vi "Config Info Put.vi"(6 "PLC Comms":T2={"PLC boolean read Tags"={"AT glass position"={"Tag Name"="S060.PXI.Signals.PlltData.SN", "Network Path"="172.15.51.1,1,0", "use opc"=FALSE, "DataSocket Reference"={"CWDSLib._DCWDataSocket"=refnum, "CWDSLib._DCWData"=refnum, "OnDataUpdated"=0, "OnStatusUpdated"=0}}, "AT shade position"={"Tag Name"="S060.PXI.Signals.PlltData.SN", "Network Path"="172.15.51.1,1,0", "use opc"=FALSE, "DataSocket Reference"={"CWDSLib._DCWDataSocket"=refnum, "CWDSLib._DCWData"=refnum, "OnDataUpdated"=0, "OnStatusUpdated"=0}}, "AT in glass wand lower pos"={"Tag Name"="S060.PXI.Signals.PlltData.SN", "Network Path"="172.15.51.1,1,0", "use opc"=FALSE, "DataSocket Reference"={"CWDSLib._DCWDataSocket"=refnum, "CWDSLib._DCWData"=refnum, "OnDataUpdated"=0, "OnStatusUpdated"=0}}, "AT in glass wand up pos"={"Tag Name"="S060.PXI.Signals.PlltData.SN", "Network Path"="172.15.51.1,1,0", "use opc"=FALSE, "DataSocket Reference"={"CWDSLib._DCWDataSocket"=refnum, "CWDSLib._DCWData"=refnum, "OnDataUpdated"=0, "OnStatusUpdated"=0}}, "AT in sunshad wand lower pos"={"Tag Name"="S060.PXI.Signals.PlltData.SN", "Network Path"="172.15.51.1,1,0", "use opc"=FALSE, "DataSocket Reference"={"CWDSLib._DCWDataSocket"=refnum, "CWDSLib._DCWData"=refnum, "OnDataUpdated"=0, "OnStatusUpdated"=0}}, "AT in sunshad wand up pos"={"Tag Name"="S060.PXI.Signals.PlltData.SN", "Network Path"="172.15.51.1,1,0", "use opc"=FALSE, "DataSocket Reference"={"CWDSLib._DCWDataSocket"=refnum, "CWDSLib._DCWData"=refnum, "OnDataUpdated"=0, "OnStatusUpdated"=0}}, "AT in wand home pos"={"Tag Name"="S060.PXI.Signals.PlltData.SN", "Network Path"="172.15.51.1,1,0", "use opc"=FALSE, "DataSocket Reference"={"CWDSLib._DCWDataSocket"=refnum, "CWDSLib._DCWData"=refnum, "OnDataUpdated"=0, "OnStatusUpdated"=0}}, "LVDT's Extended"={"Tag Name"="S060.PXI.Signals.PlltData.SN", "Network Path"="172.15.51.1,1,0", "use opc"=FALSE, "DataSocket Reference"={"CWDSLib._DCWDataSocket"=refnum, "CWDSLib._DCWData"=refnum, "OnDataUpdated"=0, "OnStatusUpdated"=0}}, "bolt check 1"={"Tag Name"="S060.PXI.Signals.PlltData.SN", "Network Path"="172.15.51.1,1,0", "use opc"=FALSE, "DataSocket Reference"={"CWDSLib._DCWDataSocket"=refnum, "CWDSLib._DCWData"=refnum, "OnDataUpdated"=0, "OnStatusUpdated"=0}}, "bolt check 2"={"Tag Name"="S060.PXI.Signals.PlltData.SN", "Network Path"="172.15.51.1,1,0", "use opc"=FALSE, "DataSocket Reference"={"CWDSLib._DCWDataSocket"=refnum, "CWDSLib._DCWData"=refnum, "OnDataUpdated"=0, "OnStatusUpdated"=0}}, "bolt check 3"={"Tag Name"="S060.PXI.Signals.PlltData.SN", "Network Path"="172.15.51.1,1,0", "use opc"=FALSE, "DataSocket Reference"={"CWDSLib._DCWDataSocket"=refnum, "CWDSLib._DCWData"=refnum, "OnDataUpdated"=0, "OnStatusUpdated"=0}}, "bolt check 4"={"Tag Name"="S060.PXI.Signals.PlltData.SN", "Network Path"="172.15.51.1,1,0", "use opc"=FALSE, "DataSocket Reference"={"CWDSLib._DCWDataSocket"=refnum, "CWDSLib._DCWData"=refnum, "OnDataUpdated"=0, "OnStatusUpdated"=0}}, "bolt check 5"={"Tag Name"="S060.PXI.Signals.PlltData.SN", "Network Path"="172.15.51.1,1,0", "use opc"=FALSE, "DataSocket Reference"={"CWDSLib._DCWDataSocket"=refnum, "CWDSLib._DCWData"=refnum, "OnDataUpdated"=0, "OnStatusUpdated"=0}}, "bolt check 6"={"Tag Name"="S060.PXI.Signals.PlltData.SN", "Network Path"="172.15.51.1,1,0", "use opc"=FALSE, "DataSocket Reference"={"CWDSLib._DCWDataSocket"=refnum, "CWDSLib._DCWData"=refnum, "OnDataUpdated"=0, "OnStatusUpdated"=0}}, "bolt check 7"={"Tag Name"="S060.PXI.Signals.PlltData.SN", "Network Path"="172.15.51.1,1,0", "use opc"=FALSE, "DataSocket Reference"={"CWDSLib._DCWDataSocket"=refnum, "CWDSLib._DCWData"=refnum, "OnDataUpdated"=0, "OnStatusUpdated"=0}}, "bolt check 8"={"Tag Name"="S060.PXI.Signals.PlltData.SN", "Network Path"="172.15.51.1,1,0", "use opc"=FALSE, "DataSocket Reference"={"CWDSLib._DCWDataSocket"=refnum, "CWDSLib._DCWData"=refnum, "OnDataUpdated"=0, "OnStatusUpdated"=0}}, "start"={"Tag Name"="S060.PXI.Signals.PlltData.SN", "Network Path"="172.15.51.1,1,0", "use opc"=FALSE, "DataSocket Reference"={"CWDSLib._DCWDataSocket"=refnum, "CWDSLib._DCWData"=refnum, "OnDataUpdated"=0, "OnStatusUpdated"=0}}, "abort"={"Tag Name"="S060.PXI.Signals.PlltData.SN", "Network Path"="172.15.51.1,1,0", "use opc"=FALSE, "DataSocket Reference"={"CWDSLib._DCWDataSocket"=refnum, "CWDSLib._DCWData"=refnum, "OnDataUpdated"=0, "OnStatusUpdated"=0}}, "LVDT's Retracted"={"Tag Name"="S060.PXI.Signals.PlltData.SN", "Network Path"="172.15.51.1,1,0", "use opc"=FALSE, "DataSocket Reference"={"CWDSLib._DCWDataSocket"=refnum, "CWDSLib._DCWData"=refnum, "OnDataUpdated"=0, "OnStatusUpdated"=0}}, "manual barcode print"={"Tag Name"="S060.PXI.Signals.PlltData.SN", "Network Path"="172.15.51.1,1,0", "use opc"=FALSE, "DataSocket Reference"={"CWDSLib._DCWDataSocket"=refnum, "CWDSLib._DCWData"=refnum, "OnDataUpdated"=0, "OnStatusUpdated"=0}}, "ss servo at open"={"Tag Name"="S060.PXI.Signals.PlltData.SN", "Network Path"="172.15.51.1,1,0", "use opc"=FALSE, "DataSocket Reference"={"CWDSLib._DCWDataSocket"=refnum, "CWDSLib._DCWData"=refnum, "OnDataUpdated"=0, "OnStatusUpdated"=0}}, "ss servo at close"={"Tag Name"="S060.PXI.Signals.PlltData.SN", "Network Path"="172.15.51.1,1,0", "use opc"=FALSE, "DataSocket Reference"={"CWDSLib._DCWDataSocket"=refnum, "CWDSLib._DCWData"=refnum, "OnDataUpdated"=0, "OnStatusUpdated"=0}}, "ss servo opening"={"Tag Name"="S060.PXI.Signals.PlltData.SN", "Network Path"="172.15.51.1,1,0", "use opc"=FALSE, "DataSocket Reference"={"CWDSLib._DCWDataSocket"=refnum, "CWDSLib._DCWData"=refnum, "OnDataUpdated"=0, "OnStatusUpdated"=0}}, "ss servo closing"={"Tag Name"="S060.PXI.Signals.PlltData.SN", "Network Path"="172.15.51.1,1,0", "use opc"=FALSE, "DataSocket Reference"={"CWDSLib._DCWDataSocket"=refnum, "CWDSLib._DCWData"=refnum, "OnDataUpdated"=0, "OnStatusUpdated"=0}}, "control slide at home"={"Tag Name"="S060.PXI.Signals.PlltData.SN", "Network Path"="172.15.51.1,1,0", "use opc"=FALSE, "DataSocket Reference"={"CWDSLib._DCWDataSocket"=refnum, "CWDSLib._DCWData"=refnum, "OnDataUpdated"=0, "OnStatusUpdated"=0}}, "control slide left good"={"Tag Name"="S060.PXI.Signals.PlltData.SN", "Network Path"="172.15.51.1,1,0", "use opc"=FALSE, "DataSocket Reference"={"CWDSLib._DCWDataSocket"=refnum, "CWDSLib._DCWData"=refnum, "OnDataUpdated"=0, "OnStatusUpdated"=0}}, "control slide left over stroke"={"Tag Name"="S060.PXI.Signals.PlltData.SN", "Network Path"="172.15.51.1,1,0", "use opc"=FALSE, "DataSocket Reference"={"CWDSLib._DCWDataSocket"=refnum, "CWDSLib._DCWData"=refnum, "OnDataUpdated"=0, "OnStatusUpdated"=0}}, "control slide right good"={"Tag Name"="S060.PXI.Signals.PlltData.SN", "Network Path"="172.15.51.1,1,0", "use opc"=FALSE, "DataSocket Reference"={"CWDSLib._DCWDataSocket"=refnum, "CWDSLib._DCWData"=refnum, "OnDataUpdated"=0, "OnStatusUpdated"=0}}, "control slide right over stroke"={"Tag Name"="S060.PXI.Signals.PlltData.SN", "Network Path"="172.15.51.1,1,0", "use opc"=FALSE, "DataSocket Reference"={"CWDSLib._DCWDataSocket"=refnum, "CWDSLib._DCWData"=refnum, "OnDataUpdated"=0, "OnStatusUpdated"=0}}, "wind deflector high speed pos"={"Tag Name"="S060.PXI.Signals.PlltData.SN", "Network Path"="172.15.51.1,1,0", "use opc"=FALSE, "DataSocket Reference"={"CWDSLib._DCWDataSocket"=refnum, "CWDSLib._DCWData"=refnum, "OnDataUpdated"=0, "OnStatusUpdated"=0}}, "wind deflector low speed pos"={"Tag Name"="S060.PXI.Signals.PlltData.SN", "Network Path"="172.15.51.1,1,0", "use opc"=FALSE, "DataSocket Reference"={"CWDSLib._DCWDataSocket"=refnum, "CWDSLib._DCWData"=refnum, "OnDataUpdated"=0, "OnStatusUpdated"=0}}, "AT VentPMACatHome"={"Tag Name"="S060.PXI.Signals.PlltData.SN", "Network Path"="172.15.51.1,1,0", "use opc"=FALSE, "DataSocket Reference"={"CWDSLib._DCWDataSocket"=refnum, "CWDSLib._DCWData"=refnum, "OnDataUpdated"=0, "OnStatusUpdated"=0}}, "AT VentPMACisExtend"={"Tag Name"="S060.PXI.Signals.PlltData.SN", "Network Path"="172.15.51.1,1,0", "use opc"=FALSE, "DataSocket Reference"={"CWDSLib._DCWDataSocket"=refnum, "CWDSLib._DCWData"=refnum, "OnDataUpdated"=0, "OnStatusUpdated"=0}}, "SS Barcode Scanner Bypassed"={"Tag Name"="S060.PXI.Signals.PlltData.SN", "Network Path"="172.15.51.1,1,0", "use opc"=FALSE, "DataSocket Reference"={"CWDSLib._DCWDataSocket"=refnum, "CWDSLib._DCWData"=refnum, "OnDataUpdated"=0, "OnStatusUpdated"=0}}, "Check Frame Barcode"={"Tag Name"="S060.PXI.Signals.PlltData.SN", "Network Path"="172.15.51.1,1,0", "use opc"=FALSE, "DataSocket Reference"={"CWDSLib._DCWDataSocket"=refnum, "CWDSLib._DCWData"=refnum, "OnDataUpdated"=0, "OnStatusUpdated"=0}}, "Z LVDTs Extended"={"Tag Name"="S060.PXI.Signals.PlltData.SN", "Network Path"="172.15.51.1,1,0", "use opc"=FALSE, "DataSocket Reference"={"CWDSLib._DCWDataSocket"=refnum, "CWDSLib._DCWData"=refnum, "OnDataUpdated"=0, "OnStatusUpdated"=0}}, "NVH Operator Pass"={"Tag Name"="S060.PXI.Signals.PlltData.SN", "Network Path"="172.15.51.1,1,0", "use opc"=FALSE, "DataSocket Reference"={"CWDSLib._DCWDataSocket"=refnum, "CWDSLib._DCWData"=refnum, "OnDataUpdated"=0, "OnStatusUpdated"=0}}, "NVH Operator Fail"={"Tag Name"="S060.PXI.Signals.PlltData.SN", "Network Path"="172.15.51.1,1,0", "use opc"=FALSE, "DataSocket Reference"={"CWDSLib._DCWDataSocket"=refnum, "CWDSLib._DCWData"=refnum, "OnDataUpdated"=0, "OnStatusUpdated"=0}}, "NVH Operator Express Glass Open"={"Tag Name"="S060.PXI.Signals.PlltData.SN", "Network Path"="172.15.51.1,1,0", "use opc"=FALSE, "DataSocket Reference"={"CWDSLib._DCWDataSocket"=refnum, "CWDSLib._DCWData"=refnum, "OnDataUpdated"=0, "OnStatusUpdated"=0}}, "NVH Operator Express Glass Close"={"Tag Name"="S060.PXI.Signals.PlltData.SN", "Network Path"="172.15.51.1,1,0", "use opc"=FALSE, "DataSocket Reference"={"CWDSLib._DCWDataSocket"=refnum, "CWDSLib._DCWData"=refnum, "OnDataUpdated"=0, "OnStatusUpdated"=0}}, "NVH Operator Express Rollo Open01"={"Tag Name"="S060.PXI.Signals.PlltData.SN", "Network Path"="172.15.51.1,1,0", "use opc"=FALSE, "DataSocket Reference"={"CWDSLib._DCWDataSocket"=refnum, "CWDSLib._DCWData"=refnum, "OnDataUpdated"=0, "OnStatusUpdated"=0}}, "NVH Operator Express Rollo Close01"={"Tag Name"="S060.PXI.Signals.PlltData.SN", "Network Path"="172.15.51.1,1,0", "use opc"=FALSE, "DataSocket Reference"={"CWDSLib._DCWDataSocket"=refnum, "CWDSLib._DCWData"=refnum, "OnDataUpdated"=0, "OnStatusUpdated"=0}}, "NVH Operator Express Rollo Open02"={"Tag Name"="S060.PXI.Signals.PlltData.SN", "Network Path"="172.15.51.1,1,0", "use opc"=FALSE, "DataSocket Reference"={"CWDSLib._DCWDataSocket"=refnum, "CWDSLib._DCWData"=refnum, "OnDataUpdated"=0, "OnStatusUpdated"=0}}, "NVH Operator Express Rollo Close02"={"Tag Name"="S060.PXI.Signals.PlltData.SN", "Network Path"="172.15.51.1,1,0", "use opc"=FALSE, "DataSocket Reference"={"CWDSLib._DCWDataSocket"=refnum, "CWDSLib._DCWData"=refnum, "OnDataUpdated"=0, "OnStatusUpdated"=0}}, "NVH Operator Vent Open Noise"={"Tag Name"="S060.PXI.Signals.PlltData.SN", "Network Path"="172.15.51.1,1,0", "use opc"=FALSE, "DataSocket Reference"={"CWDSLib._DCWDataSocket"=refnum, "CWDSLib._DCWData"=refnum, "OnDataUpdated"=0, "OnStatusUpdated"=0}}, "NVH Operator Vent Close Noise"={"Tag Name"="S060.PXI.Signals.PlltData.SN", "Network Path"="172.15.51.1,1,0", "use opc"=FALSE, "DataSocket Reference"={"CWDSLib._DCWDataSocket"=refnum, "CWDSLib._DCWData"=refnum, "OnDataUpdated"=0, "OnStatusUpdated"=0}}, "NVH Operator Sunshade Open Noise"={"Tag Name"="S060.PXI.Signals.PlltData.SN", "Network Path"="172.15.51.1,1,0", "use opc"=FALSE, "DataSocket Reference"={"CWDSLib._DCWDataSocket"=refnum, "CWDSLib._DCWData"=refnum, "OnDataUpdated"=0, "OnStatusUpdated"=0}}, "NVH Operator Sunshade Close Noise"={"Tag Name"="S060.PXI.Signals.PlltData.SN", "Network Path"="172.15.51.1,1,0", "use opc"=FALSE, "DataSocket Reference"={"CWDSLib._DCWDataSocket"=refnum, "CWDSLib._DCWData"=refnum, "OnDataUpdated"=0, "OnStatusUpdated"=0}}, "NVH Operator Glass Open Noise"={"Tag Name"="S060.PXI.Signals.PlltData.SN", "Network Path"="172.15.51.1,1,0", "use opc"=FALSE, "DataSocket Reference"={"CWDSLib._DCWDataSocket"=refnum, "CWDSLib._DCWData"=refnum, "OnDataUpdated"=0, "OnStatusUpdated"=0}}, "NVH Operator Glass Close Noise"={"Tag Name"="S060.PXI.Signals.PlltData.SN", "Network Path"="172.15.51.1,1,0", "use opc"=FALSE, "DataSocket Reference"={"CWDSLib._DCWDataSocket"=refnum, "CWDSLib._DCWData"=refnum, "OnDataUpdated"=0, "OnStatusUpdated"=0}}, "NVH Operator Finish"={"Tag Name"="S060.PXI.Signals.PlltData.SN", "Network Path"="172.15.51.1,1,0", "use opc"=FALSE, "DataSocket Reference"={"CWDSLib._DCWDataSocket"=refnum, "CWDSLib._DCWData"=refnum, "OnDataUpdated"=0, "OnStatusUpdated"=0}}, "NVH Operator Check"={"Tag Name"="S060.PXI.Signals.PlltData.SN", "Network Path"="172.15.51.1,1,0", "use opc"=FALSE, "DataSocket Reference"={"CWDSLib._DCWDataSocket"=refnum, "CWDSLib._DCWData"=refnum, "OnDataUpdated"=0, "OnStatusUpdated"=0}}, "windproof position"={"Tag Name"="S060.PXI.Signals.PlltData.SN", "Network Path"="172.15.51.1,1,0", "use opc"=FALSE, "DataSocket Reference"={"CWDSLib._DCWDataSocket"=refnum, "CWDSLib._DCWData"=refnum, "OnDataUpdated"=0, "OnStatusUpdated"=0}}, "NVH Operator Express Glass vent Open"={"Tag Name"="S060.PXI.Signals.PlltData.SN", "Network Path"="172.15.51.1,1,0", "use opc"=FALSE, "DataSocket Reference"={"CWDSLib._DCWDataSocket"=refnum, "CWDSLib._DCWData"=refnum, "OnDataUpdated"=0, "OnStatusUpdated"=0}}, "NVH Operator Express Glass Vent Close"={"Tag Name"="S060.PXI.Signals.PlltData.SN", "Network Path"="172.15.51.1,1,0", "use opc"=FALSE, "DataSocket Reference"={"CWDSLib._DCWDataSocket"=refnum, "CWDSLib._DCWData"=refnum, "OnDataUpdated"=0, "OnStatusUpdated"=0}}, "NVH Operator Re-do"={"Tag Name"="S060.PXI.Signals.PlltData.SN", "Network Path"="172.15.51.1,1,0", "use opc"=FALSE, "DataSocket Reference"={"CWDSLib._DCWDataSocket"=refnum, "CWDSLib._DCWData"=refnum, "OnDataUpdated"=0, "OnStatusUpdated"=0}}, "AT at vent ATS test pos"={"Tag Name"="S060.PXI.Signals.PlltData.SN", "Network Path"="172.15.51.1,1,0", "use opc"=FALSE, "DataSocket Reference"={"CWDSLib._DCWDataSocket"=refnum, "CWDSLib._DCWData"=refnum, "OnDataUpdated"=0, "OnStatusUpdated"=0}}, "AT at vent ATS Home pos"={"Tag Name"="S060.PXI.Signals.PlltData.SN", "Network Path"="172.15.51.1,1,0", "use opc"=FALSE, "DataSocket Reference"={"CWDSLib._DCWDataSocket"=refnum, "CWDSLib._DCWData"=refnum, "OnDataUpdated"=0, "OnStatusUpdated"=0}}, "Start Adjust LVDT"={"Tag Name"="S060.PXI.Signals.PlltData.SN", "Network Path"="172.15.51.1,1,0", "use opc"=FALSE, "DataSocket Reference"={"CWDSLib._DCWDataSocket"=refnum, "CWDSLib._DCWData"=refnum, "OnDataUpdated"=0, "OnStatusUpdated"=0}}, "Finish Adjust LVDT"={"Tag Name"="S060.PXI.Signals.PlltData.SN", "Network Path"="172.15.51.1,1,0", "use opc"=FALSE, "DataSocket Reference"={"CWDSLib._DCWDataSocket"=refnum, "CWDSLib._DCWData"=refnum, "OnDataUpdated"=0, "OnStatusUpdated"=0}}}, "PLC bool write Tags"={"AT set glass wand lower"={"Tag Name"="S060.PXI.Signals.PlltData.SN", "Network Path"="172.15.51.1,1,0", "use opc"=FALSE, "DataSocket Reference"={"CWDSLib._DCWDataSocket"=refnum, "CWDSLib._DCWData"=refnum, "OnDataUpdated"=0, "OnStatusUpdated"=0}}, "AT set sunshade wand lower"={"Tag Name"="S060.PXI.Signals.PlltData.SN", "Network Path"="172.15.51.1,1,0", "use opc"=FALSE, "DataSocket Reference"={"CWDSLib._DCWDataSocket"=refnum, "CWDSLib._DCWData"=refnum, "OnDataUpdated"=0, "OnStatusUpdated"=0}}, "AT set sunshade wand up"={"Tag Name"="S060.PXI.Signals.PlltData.SN", "Network Path"="172.15.51.1,1,0", "use opc"=FALSE, "DataSocket Reference"={"CWDSLib._DCWDataSocket"=refnum, "CWDSLib._DCWData"=refnum, "OnDataUpdated"=0, "OnStatusUpdated"=0}}, "AT set glass wand up"={"Tag Name"="S060.PXI.Signals.PlltData.SN", "Network Path"="172.15.51.1,1,0", "use opc"=FALSE, "DataSocket Reference"={"CWDSLib._DCWDataSocket"=refnum, "CWDSLib._DCWData"=refnum, "OnDataUpdated"=0, "OnStatusUpdated"=0}}, "AT set wand home pos"={"Tag Name"="S060.PXI.Signals.PlltData.SN", "Network Path"="172.15.51.1,1,0", "use opc"=FALSE, "DataSocket Reference"={"CWDSLib._DCWDataSocket"=refnum, "CWDSLib._DCWData"=refnum, "OnDataUpdated"=0, "OnStatusUpdated"=0}}, "Test Complete Pass"={"Tag Name"="S060.PXI.Signals.PlltData.SN", "Network Path"="172.15.51.1,1,0", "use opc"=FALSE, "DataSocket Reference"={"CWDSLib._DCWDataSocket"=refnum, "CWDSLib._DCWData"=refnum, "OnDataUpdated"=0, "OnStatusUpdated"=0}}, "Test Complete Fail"={"Tag Name"="S060.PXI.Signals.PlltData.SN", "Network Path"="172.15.51.1,1,0", "use opc"=FALSE, "DataSocket Reference"={"CWDSLib._DCWDataSocket"=refnum, "CWDSLib._DCWData"=refnum, "OnDataUpdated"=0, "OnStatusUpdated"=0}}, "Test Started"={"Tag Name"="S060.PXI.Signals.PlltData.SN", "Network Path"="172.15.51.1,1,0", "use opc"=FALSE, "DataSocket Reference"={"CWDSLib._DCWDataSocket"=refnum, "CWDSLib._DCWData"=refnum, "OnDataUpdated"=0, "OnStatusUpdated"=0}}, "Retract LVDT's"={"Tag Name"="S060.PXI.Signals.PlltData.SN", "Network Path"="172.15.51.1,1,0", "use opc"=FALSE, "DataSocket Reference"={"CWDSLib._DCWDataSocket"=refnum, "CWDSLib._DCWData"=refnum, "OnDataUpdated"=0, "OnStatusUpdated"=0}}, "Extend LVDT's"={"Tag Name"="S060.PXI.Signals.PlltData.SN", "Network Path"="172.15.51.1,1,0", "use opc"=FALSE, "DataSocket Reference"={"CWDSLib._DCWDataSocket"=refnum, "CWDSLib._DCWData"=refnum, "OnDataUpdated"=0, "OnStatusUpdated"=0}}, "ss servo open"={"Tag Name"="S060.PXI.Signals.PlltData.SN", "Network Path"="172.15.51.1,1,0", "use opc"=FALSE, "DataSocket Reference"={"CWDSLib._DCWDataSocket"=refnum, "CWDSLib._DCWData"=refnum, "OnDataUpdated"=0, "OnStatusUpdated"=0}}, "ss servo close"={"Tag Name"="S060.PXI.Signals.PlltData.SN", "Network Path"="172.15.51.1,1,0", "use opc"=FALSE, "DataSocket Reference"={"CWDSLib._DCWDataSocket"=refnum, "CWDSLib._DCWData"=refnum, "OnDataUpdated"=0, "OnStatusUpdated"=0}}, "control slide start"={"Tag Name"="S060.PXI.Signals.PlltData.SN", "Network Path"="172.15.51.1,1,0", "use opc"=FALSE, "DataSocket Reference"={"CWDSLib._DCWDataSocket"=refnum, "CWDSLib._DCWData"=refnum, "OnDataUpdated"=0, "OnStatusUpdated"=0}}, "control slide stop"={"Tag Name"="S060.PXI.Signals.PlltData.SN", "Network Path"="172.15.51.1,1,0", "use opc"=FALSE, "DataSocket Reference"={"CWDSLib._DCWDataSocket"=refnum, "CWDSLib._DCWData"=refnum, "OnDataUpdated"=0, "OnStatusUpdated"=0}}, "AT VentPMACHome"={"Tag Name"="S060.PXI.Signals.PlltData.SN", "Network Path"="172.15.51.1,1,0", "use opc"=FALSE, "DataSocket Reference"={"CWDSLib._DCWDataSocket"=refnum, "CWDSLib._DCWData"=refnum, "OnDataUpdated"=0, "OnStatusUpdated"=0}}, "AT VentPMACExtended"={"Tag Name"="S060.PXI.Signals.PlltData.SN", "Network Path"="172.15.51.1,1,0", "use opc"=FALSE, "DataSocket Reference"={"CWDSLib._DCWDataSocket"=refnum, "CWDSLib._DCWData"=refnum, "OnDataUpdated"=0, "OnStatusUpdated"=0}}, "Good Frame Barcode"={"Tag Name"="S060.PXI.Signals.PlltData.SN", "Network Path"="172.15.51.1,1,0", "use opc"=FALSE, "DataSocket Reference"={"CWDSLib._DCWDataSocket"=refnum, "CWDSLib._DCWData"=refnum, "OnDataUpdated"=0, "OnStatusUpdated"=0}}, "Bad Frame Barcode"={"Tag Name"="S060.PXI.Signals.PlltData.SN", "Network Path"="172.15.51.1,1,0", "use opc"=FALSE, "DataSocket Reference"={"CWDSLib._DCWDataSocket"=refnum, "CWDSLib._DCWData"=refnum, "OnDataUpdated"=0, "OnStatusUpdated"=0}}, "Extend Z LVDTS"={"Tag Name"="S060.PXI.Signals.PlltData.SN", "Network Path"="172.15.51.1,1,0", "use opc"=FALSE, "DataSocket Reference"={"CWDSLib._DCWDataSocket"=refnum, "CWDSLib._DCWData"=refnum, "OnDataUpdated"=0, "OnStatusUpdated"=0}}, "NVH SunRoof Moving"={"Tag Name"="S060.PXI.Signals.PlltData.SN", "Network Path"="172.15.51.1,1,0", "use opc"=FALSE, "DataSocket Reference"={"CWDSLib._DCWDataSocket"=refnum, "CWDSLib._DCWData"=refnum, "OnDataUpdated"=0, "OnStatusUpdated"=0}}, "NVH SunRoof Stop"={"Tag Name"="S060.PXI.Signals.PlltData.SN", "Network Path"="172.15.51.1,1,0", "use opc"=FALSE, "DataSocket Reference"={"CWDSLib._DCWDataSocket"=refnum, "CWDSLib._DCWData"=refnum, "OnDataUpdated"=0, "OnStatusUpdated"=0}}, "NVH Pass"={"Tag Name"="S060.PXI.Signals.PlltData.SN", "Network Path"="172.15.51.1,1,0", "use opc"=FALSE, "DataSocket Reference"={"CWDSLib._DCWDataSocket"=refnum, "CWDSLib._DCWData"=refnum, "OnDataUpdated"=0, "OnStatusUpdated"=0}}, "NVH Fail"={"Tag Name"="S060.PXI.Signals.PlltData.SN", "Network Path"="172.15.51.1,1,0", "use opc"=FALSE, "DataSocket Reference"={"CWDSLib._DCWDataSocket"=refnum, "CWDSLib._DCWData"=refnum, "OnDataUpdated"=0, "OnStatusUpdated"=0}}, "NVH Operator Express Glass Opened"={"Tag Name"="S060.PXI.Signals.PlltData.SN", "Network Path"="172.15.51.1,1,0", "use opc"=FALSE, "DataSocket Reference"={"CWDSLib._DCWDataSocket"=refnum, "CWDSLib._DCWData"=refnum, "OnDataUpdated"=0, "OnStatusUpdated"=0}}, "NVH Operator Express Glass Closed"={"Tag Name"="S060.PXI.Signals.PlltData.SN", "Network Path"="172.15.51.1,1,0", "use opc"=FALSE, "DataSocket Reference"={"CWDSLib._DCWDataSocket"=refnum, "CWDSLib._DCWData"=refnum, "OnDataUpdated"=0, "OnStatusUpdated"=0}}, "NVH Operator Express Rollo Opened01"={"Tag Name"="S060.PXI.Signals.PlltData.SN", "Network Path"="172.15.51.1,1,0", "use opc"=FALSE, "DataSocket Reference"={"CWDSLib._DCWDataSocket"=refnum, "CWDSLib._DCWData"=refnum, "OnDataUpdated"=0, "OnStatusUpdated"=0}}, "NVH Operator Express Rollo Closed01"={"Tag Name"="S060.PXI.Signals.PlltData.SN", "Network Path"="172.15.51.1,1,0", "use opc"=FALSE, "DataSocket Reference"={"CWDSLib._DCWDataSocket"=refnum, "CWDSLib._DCWData"=refnum, "OnDataUpdated"=0, "OnStatusUpdated"=0}}, "NVH Operator Express Rollo Opened02"={"Tag Name"="S060.PXI.Signals.PlltData.SN", "Network Path"="172.15.51.1,1,0", "use opc"=FALSE, "DataSocket Reference"={"CWDSLib._DCWDataSocket"=refnum, "CWDSLib._DCWData"=refnum, "OnDataUpdated"=0, "OnStatusUpdated"=0}}, "NVH Operator Pass"={"Tag Name"="S060.PXI.Signals.PlltData.SN", "Network Path"="172.15.51.1,1,0", "use opc"=FALSE, "DataSocket Reference"={"CWDSLib._DCWDataSocket"=refnum, "CWDSLib._DCWData"=refnum, "OnDataUpdated"=0, "OnStatusUpdated"=0}}, "NVH Operator Fail"={"Tag Name"="S060.PXI.Signals.PlltData.SN", "Network Path"="172.15.51.1,1,0", "use opc"=FALSE, "DataSocket Reference"={"CWDSLib._DCWDataSocket"=refnum, "CWDSLib._DCWData"=refnum, "OnDataUpdated"=0, "OnStatusUpdated"=0}}, "NVH Operator Check"={"Tag Name"="S060.PXI.Signals.PlltData.SN", "Network Path"="172.15.51.1,1,0", "use opc"=FALSE, "DataSocket Reference"={"CWDSLib._DCWDataSocket"=refnum, "CWDSLib._DCWData"=refnum, "OnDataUpdated"=0, "OnStatusUpdated"=0}}, "NVH Operator Vent Open Noise"={"Tag Name"="S060.PXI.Signals.PlltData.SN", "Network Path"="172.15.51.1,1,0", "use opc"=FALSE, "DataSocket Reference"={"CWDSLib._DCWDataSocket"=refnum, "CWDSLib._DCWData"=refnum, "OnDataUpdated"=0, "OnStatusUpdated"=0}}, "NVH Operator Vent Close Noise"={"Tag Name"="S060.PXI.Signals.PlltData.SN", "Network Path"="172.15.51.1,1,0", "use opc"=FALSE, "DataSocket Reference"={"CWDSLib._DCWDataSocket"=refnum, "CWDSLib._DCWData"=refnum, "OnDataUpdated"=0, "OnStatusUpdated"=0}}, "NVH Operator Sunshade Open Noise"={"Tag Name"="S060.PXI.Signals.PlltData.SN", "Network Path"="172.15.51.1,1,0", "use opc"=FALSE, "DataSocket Reference"={"CWDSLib._DCWDataSocket"=refnum, "CWDSLib._DCWData"=refnum, "OnDataUpdated"=0, "OnStatusUpdated"=0}}, "NVH Operator Sunshade Close Noise"={"Tag Name"="S060.PXI.Signals.PlltData.SN", "Network Path"="172.15.51.1,1,0", "use opc"=FALSE, "DataSocket Reference"={"CWDSLib._DCWDataSocket"=refnum, "CWDSLib._DCWData"=refnum, "OnDataUpdated"=0, "OnStatusUpdated"=0}}, "NVH Operator Glass Open Noise"={"Tag Name"="S060.PXI.Signals.PlltData.SN", "Network Path"="172.15.51.1,1,0", "use opc"=FALSE, "DataSocket Reference"={"CWDSLib._DCWDataSocket"=refnum, "CWDSLib._DCWData"=refnum, "OnDataUpdated"=0, "OnStatusUpdated"=0}}, "NVH Operator Glass Close Noise"={"Tag Name"="S060.PXI.Signals.PlltData.SN", "Network Path"="172.15.51.1,1,0", "use opc"=FALSE, "DataSocket Reference"={"CWDSLib._DCWDataSocket"=refnum, "CWDSLib._DCWData"=refnum, "OnDataUpdated"=0, "OnStatusUpdated"=0}}, "NVH Operator Finish"={"Tag Name"="S060.PXI.Signals.PlltData.SN", "Network Path"="172.15.51.1,1,0", "use opc"=FALSE, "DataSocket Reference"={"CWDSLib._DCWDataSocket"=refnum, "CWDSLib._DCWData"=refnum, "OnDataUpdated"=0, "OnStatusUpdated"=0}}, "Barcode01 OK"={"Tag Name"="S060.PXI.Signals.PlltData.SN", "Network Path"="172.15.51.1,1,0", "use opc"=FALSE, "DataSocket Reference"={"CWDSLib._DCWDataSocket"=refnum, "CWDSLib._DCWData"=refnum, "OnDataUpdated"=0, "OnStatusUpdated"=0}}, "Barcode02 OK"={"Tag Name"="S060.PXI.Signals.PlltData.SN", "Network Path"="172.15.51.1,1,0", "use opc"=FALSE, "DataSocket Reference"={"CWDSLib._DCWDataSocket"=refnum, "CWDSLib._DCWData"=refnum, "OnDataUpdated"=0, "OnStatusUpdated"=0}}, "AT set to Vent ATS Test Pos"={"Tag Name"="S060.PXI.Signals.PlltData.SN", "Network Path"="172.15.51.1,1,0", "use opc"=FALSE, "DataSocket Reference"={"CWDSLib._DCWDataSocket"=refnum, "CWDSLib._DCWData"=refnum, "OnDataUpdated"=0, "OnStatusUpdated"=0}}, "AT set to Vent ATS Home Pos"={"Tag Name"="S060.PXI.Signals.PlltData.SN", "Network Path"="172.15.51.1,1,0", "use opc"=FALSE, "DataSocket Reference"={"CWDSLib._DCWDataSocket"=refnum, "CWDSLib._DCWData"=refnum, "OnDataUpdated"=0, "OnStatusUpdated"=0}}, "Move LVDT Adjust Station"={"Tag Name"="S060.PXI.Signals.PlltData.SN", "Network Path"="172.15.51.1,1,0", "use opc"=FALSE, "DataSocket Reference"={"CWDSLib._DCWDataSocket"=refnum, "CWDSLib._DCWData"=refnum, "OnDataUpdated"=0, "OnStatusUpdated"=0}}}, "PLC string read Tags"={"Serial Number"={"Tag Name"="S060.PXI.Signals.PlltData.SN", "Network Path"="172.15.51.1,1,0", "use opc"=FALSE, "DataSocket Reference"={"CWDSLib._DCWDataSocket"=refnum, "CWDSLib._DCWData"=refnum, "OnDataUpdated"=0, "OnStatusUpdated"=0}}, "Pallet Number"={"Tag Name"="S060.PXI.Signals.PlltData.SN", "Network Path"="172.15.51.1,1,0", "use opc"=FALSE, "DataSocket Reference"={"CWDSLib._DCWDataSocket"=refnum, "CWDSLib._DCWData"=refnum, "OnDataUpdated"=0, "OnStatusUpdated"=0}}, "Inalfa Part Number"={"Tag Name"="S060.PXI.Signals.PlltData.SN", "Network Path"="172.15.51.1,1,0", "use opc"=FALSE, "DataSocket Reference"={"CWDSLib._DCWDataSocket"=refnum, "CWDSLib._DCWData"=refnum, "OnDataUpdated"=0, "OnStatusUpdated"=0}}, "Shade Color"={"Tag Name"="S060.PXI.Signals.PlltData.SN", "Network Path"="172.15.51.1,1,0", "use opc"=FALSE, "DataSocket Reference"={"CWDSLib._DCWDataSocket"=refnum, "CWDSLib._DCWData"=refnum, "OnDataUpdated"=0, "OnStatusUpdated"=0}}, "Model Type"={"Tag Name"="S060.PXI.Signals.PlltData.SN", "Network Path"="172.15.51.1,1,0", "use opc"=FALSE, "DataSocket Reference"={"CWDSLib._DCWDataSocket"=refnum, "CWDSLib._DCWData"=refnum, "OnDataUpdated"=0, "OnStatusUpdated"=0}}, "Customer Number"={"Tag Name"="S060.PXI.Signals.PlltData.SN", "Network Path"="172.15.51.1,1,0", "use opc"=FALSE, "DataSocket Reference"={"CWDSLib._DCWDataSocket"=refnum, "CWDSLib._DCWData"=refnum, "OnDataUpdated"=0, "OnStatusUpdated"=0}}, "Part History Number"={"Tag Name"="S060.PXI.Signals.PlltData.SN", "Network Path"="172.15.51.1,1,0", "use opc"=FALSE, "DataSocket Reference"={"CWDSLib._DCWDataSocket"=refnum, "CWDSLib._DCWData"=refnum, "OnDataUpdated"=0, "OnStatusUpdated"=0}}, "Shade 1 Barcode"={"Tag Name"="S060.PXI.Signals.PlltData.SN", "Network Path"="172.15.51.1,1,0", "use opc"=FALSE, "DataSocket Reference"={"CWDSLib._DCWDataSocket"=refnum, "CWDSLib._DCWData"=refnum, "OnDataUpdated"=0, "OnStatusUpdated"=0}}, "Shade 2 Barcode"={"Tag Name"="S060.PXI.Signals.PlltData.SN", "Network Path"="172.15.51.1,1,0", "use opc"=FALSE, "DataSocket Reference"={"CWDSLib._DCWDataSocket"=refnum, "CWDSLib._DCWData"=refnum, "OnDataUpdated"=0, "OnStatusUpdated"=0}}, "Manual Serial Number"={"Tag Name"="S060.PXI.Signals.PlltData.SN", "Network Path"="172.15.51.1,1,0", "use opc"=FALSE, "DataSocket Reference"={"CWDSLib._DCWDataSocket"=refnum, "CWDSLib._DCWData"=refnum, "OnDataUpdated"=0, "OnStatusUpdated"=0}}, "Manual Inalfa Part Number"={"Tag Name"="S060.PXI.Signals.PlltData.SN", "Network Path"="172.15.51.1,1,0", "use opc"=FALSE, "DataSocket Reference"={"CWDSLib._DCWDataSocket"=refnum, "CWDSLib._DCWData"=refnum, "OnDataUpdated"=0, "OnStatusUpdated"=0}}, "Manual Shade Color"={"Tag Name"="S060.PXI.Signals.PlltData.SN", "Network Path"="172.15.51.1,1,0", "use opc"=FALSE, "DataSocket Reference"={"CWDSLib._DCWDataSocket"=refnum, "CWDSLib._DCWData"=refnum, "OnDataUpdated"=0, "OnStatusUpdated"=0}}, "Manual Model Type"={"Tag Name"="S060.PXI.Signals.PlltData.SN", "Network Path"="172.15.51.1,1,0", "use opc"=FALSE, "DataSocket Reference"={"CWDSLib._DCWDataSocket"=refnum, "CWDSLib._DCWData"=refnum, "OnDataUpdated"=0, "OnStatusUpdated"=0}}, "Manual Customer Number"={"Tag Name"="S060.PXI.Signals.PlltData.SN", "Network Path"="172.15.51.1,1,0", "use opc"=FALSE, "DataSocket Reference"={"CWDSLib._DCWDataSocket"=refnum, "CWDSLib._DCWData"=refnum, "OnDataUpdated"=0, "OnStatusUpdated"=0}}, "Manual Part History Number"={"Tag Name"="S060.PXI.Signals.PlltData.SN", "Network Path"="172.15.51.1,1,0", "use opc"=FALSE, "DataSocket Reference"={"CWDSLib._DCWDataSocket"=refnum, "CWDSLib._DCWData"=refnum, "OnDataUpdated"=0, "OnStatusUpdated"=0}}}, "PLC string write Tags"={"barcode station error"={"Tag Name"="S060.PXI.Signals.PlltData.SN", "Network Path"="172.15.51.1,1,0", "use opc"=FALSE, "DataSocket Reference"={"CWDSLib._DCWDataSocket"=refnum, "CWDSLib._DCWData"=refnum, "OnDataUpdated"=0, "OnStatusUpdated"=0}}, "error message 0"={"Tag Name"="S060.PXI.Signals.PlltData.SN", "Network Path"="172.15.51.1,1,0", "use opc"=FALSE, "DataSocket Reference"={"CWDSLib._DCWDataSocket"=refnum, "CWDSLib._DCWData"=refnum, "OnDataUpdated"=0, "OnStatusUpdated"=0}}, "error message 1"={"Tag Name"="S060.PXI.Signals.PlltData.SN", "Network Path"="172.15.51.1,1,0", "use opc"=FALSE, "DataSocket Reference"={"CWDSLib._DCWDataSocket"=refnum, "CWDSLib._DCWData"=refnum, "OnDataUpdated"=0, "OnStatusUpdated"=0}}, "error message 2"={"Tag Name"="S060.PXI.Signals.PlltData.SN", "Network Path"="172.15.51.1,1,0", "use opc"=FALSE, "DataSocket Reference"={"CWDSLib._DCWDataSocket"=refnum, "CWDSLib._DCWData"=refnum, "OnDataUpdated"=0, "OnStatusUpdated"=0}}, "error message 3"={"Tag Name"="S060.PXI.Signals.PlltData.SN", "Network Path"="172.15.51.1,1,0", "use opc"=FALSE, "DataSocket Reference"={"CWDSLib._DCWDataSocket"=refnum, "CWDSLib._DCWData"=refnum, "OnDataUpdated"=0, "OnStatusUpdated"=0}}}, "use opc"=FALSE, "PLC/OPC Path"=""} {"PLC string write Tags"."error message 3"."DataSocket Reference"."OnStatusUpdated" format="%.0x"; "PLC string write Tags"."error message 3"."DataSocket Reference"."OnDataUpdated" format="%.0x"; "PLC string write Tags"."error message 2"."DataSocket Reference"."OnStatusUpdated" format="%.0x"; "PLC string write Tags"."error message 2"."DataSocket Reference"."OnDataUpdated" format="%.0x"; "PLC string write Tags"."error message 1"."DataSocket Reference"."OnStatusUpdated" format="%.0x"; "PLC string write Tags"."error message 1"."DataSocket Reference"."OnDataUpdated" format="%.0x"; "PLC string write Tags"."error message 0"."DataSocket Reference"."OnStatusUpdated" format="%.0x"; "PLC string write Tags"."error message 0"."DataSocket Reference"."OnDataUpdated" format="%.0x"; "PLC string write Tags"."barcode station error"."DataSocket Reference"."OnStatusUpdated" format="%.0x"; "PLC string write Tags"."barcode station error"."DataSocket Reference"."OnDataUpdated" format="%.0x"; "PLC string read Tags"."Manual Part History Number"."DataSocket Reference"."OnStatusUpdated" format="%.0x"; "PLC string read Tags"."Manual Part History Number"."DataSocket Reference"."OnDataUpdated" format="%.0x"; "PLC string read Tags"."Manual Customer Number"."DataSocket Reference"."OnStatusUpdated" format="%.0x"; "PLC string read Tags"."Manual Customer Number"."DataSocket Reference"."OnDataUpdated" format="%.0x"; "PLC string read Tags"."Manual Model Type"."DataSocket Reference"."OnStatusUpdated" format="%.0x"; "PLC string read Tags"."Manual Model Type"."DataSocket Reference"."OnDataUpdated" format="%.0x"; "PLC string read Tags"."Manual Shade Color"."DataSocket Reference"."OnStatusUpdated" format="%.0x"; "PLC string read Tags"."Manual Shade Color"."DataSocket Reference"."OnDataUpdated" format="%.0x"; "PLC string read Tags"."Manual Inalfa Part Number"."DataSocket Reference"."OnStatusUpdated" format="%.0x"; "PLC string read Tags"."Manual Inalfa Part Number"."DataSocket Reference"."OnDataUpdated" format="%.0x"; "PLC string read Tags"."Manual Serial Number"."DataSocket Reference"."OnStatusUpdated" format="%.0x"; "PLC string read Tags"."Manual Serial Number"."DataSocket Reference"."OnDataUpdated" format="%.0x"; "PLC string read Tags"."Shade 2 Barcode"."DataSocket Reference"."OnStatusUpdated" format="%.0x"; "PLC string read Tags"."Shade 2 Barcode"."DataSocket Reference"."OnDataUpdated" format="%.0x"; "PLC string read Tags"."Shade 1 Barcode"."DataSocket Reference"."OnStatusUpdated" format="%.0x"; "PLC string read Tags"."Shade 1 Barcode"."DataSocket Reference"."OnDataUpdated" format="%.0x"; "PLC string read Tags"."Part History Number"."DataSocket Reference"."OnStatusUpdated" format="%.0x"; "PLC string read Tags"."Part History Number"."DataSocket Reference"."OnDataUpdated" format="%.0x"; "PLC string read Tags"."Customer Number"."DataSocket Reference"."OnStatusUpdated" format="%.0x"; "PLC string read Tags"."Customer Number"."DataSocket Reference"."OnDataUpdated" format="%.0x"; "PLC string read Tags"."Model Type"."DataSocket Reference"."OnStatusUpdated" format="%.0x"; "PLC string read Tags"."Model Type"."DataSocket Reference"."OnDataUpdated" format="%.0x"; "PLC string read Tags"."Shade Color"."DataSocket Reference"."OnStatusUpdated" format="%.0x"; "PLC string read Tags"."Shade Color"."DataSocket Reference"."OnDataUpdated" format="%.0x"; "PLC string read Tags"."Inalfa Part Number"."DataSocket Reference"."OnStatusUpdated" format="%.0x"; "PLC string read Tags"."Inalfa Part Number"."DataSocket Reference"."OnDataUpdated" format="%.0x"; "PLC string read Tags"."Pallet Number"."DataSocket Reference"."OnStatusUpdated" format="%.0x"; "PLC string read Tags"."Pallet Number"."DataSocket Reference"."OnDataUpdated" format="%.0x"; "PLC string read Tags"."Serial Number"."DataSocket Reference"."OnStatusUpdated" format="%.0x"; "PLC string read Tags"."Serial Number"."DataSocket Reference"."OnDataUpdated" format="%.0x"; "PLC bool write Tags"."Move LVDT Adjust Station"."DataSocket Reference"."OnStatusUpdated" format="%.0x"; "PLC bool write Tags"."Move LVDT Adjust Station"."DataSocket Reference"."OnDataUpdated" format="%.0x"; "PLC bool write Tags"."AT set to Vent ATS Home Pos"."DataSocket Reference"."OnStatusUpdated" format="%.0x"; "PLC bool write Tags"."AT set to Vent ATS Home Pos"."DataSocket Reference"."OnDataUpdated" format="%.0x"; "PLC bool write Tags"."AT set to Vent ATS Test Pos"."DataSocket Reference"."OnStatusUpdated" format="%.0x"; "PLC bool write Tags"."AT set to Vent ATS Test Pos"."DataSocket Reference"."OnDataUpdated" format="%.0x"; "PLC bool write Tags"."Barcode02 OK"."DataSocket Reference"."OnStatusUpdated" format="%.0x"; "PLC bool write Tags"."Barcode02 OK"."DataSocket Reference"."OnDataUpdated" format="%.0x"; "PLC bool write Tags"."Barcode01 OK"."DataSocket Reference"."OnStatusUpdated" format="%.0x"; "PLC bool write Tags"."Barcode01 OK"."DataSocket Reference"."OnDataUpdated" format="%.0x"; "PLC bool write Tags"."AT set glass wand up"."DataSocket Reference"."OnStatusUpdated" format="%.0x"; "PLC bool write Tags"."AT set glass wand up"."DataSocket Reference"."OnDataUpdated" format="%.0x"; "PLC bool write Tags"."AT set sunshade wand up"."DataSocket Reference"."OnStatusUpdated" format="%.0x"; "PLC bool write Tags"."AT set sunshade wand up"."DataSocket Reference"."OnDataUpdated" format="%.0x"; "PLC bool write Tags"."NVH Operator Finish"."DataSocket Reference"."OnStatusUpdated" format="%.0x"; "PLC bool write Tags"."NVH Operator Finish"."DataSocket Reference"."OnDataUpdated" format="%.0x"; "PLC bool write Tags"."NVH Operator Glass Close Noise"."DataSocket Reference"."OnStatusUpdated" format="%.0x"; "PLC bool write Tags"."NVH Operator Glass Close Noise"."DataSocket Reference"."OnDataUpdated" format="%.0x"; "PLC bool write Tags"."NVH Operator Glass Open Noise"."DataSocket Reference"."OnStatusUpdated" format="%.0x"; "PLC bool write Tags"."NVH Operator Glass Open Noise"."DataSocket Reference"."OnDataUpdated" format="%.0x"; "PLC bool write Tags"."NVH Operator Sunshade Close Noise"."DataSocket Reference"."OnStatusUpdated" format="%.0x"; "PLC bool write Tags"."NVH Operator Sunshade Close Noise"."DataSocket Reference"."OnDataUpdated" format="%.0x"; "PLC bool write Tags"."NVH Operator Sunshade Open Noise"."DataSocket Reference"."OnStatusUpdated" format="%.0x"; "PLC bool write Tags"."NVH Operator Sunshade Open Noise"."DataSocket Reference"."OnDataUpdated" format="%.0x"; "PLC bool write Tags"."NVH Operator Vent Close Noise"."DataSocket Reference"."OnStatusUpdated" format="%.0x"; "PLC bool write Tags"."NVH Operator Vent Close Noise"."DataSocket Reference"."OnDataUpdated" format="%.0x"; "PLC bool write Tags"."NVH Operator Vent Open Noise"."DataSocket Reference"."OnStatusUpdated" format="%.0x"; "PLC bool write Tags"."NVH Operator Vent Open Noise"."DataSocket Reference"."OnDataUpdated" format="%.0x"; "PLC bool write Tags"."NVH Operator Check"."DataSocket Reference"."OnStatusUpdated" format="%.0x"; "PLC bool write Tags"."NVH Operator Check"."DataSocket Reference"."OnDataUpdated" format="%.0x"; "PLC bool write Tags"."NVH Operator Fail"."DataSocket Reference"."OnStatusUpdated" format="%.0x"; "PLC bool write Tags"."NVH Operator Fail"."DataSocket Reference"."OnDataUpdated" format="%.0x"; "PLC bool write Tags"."NVH Operator Pass"."DataSocket Reference"."OnStatusUpdated" format="%.0x"; "PLC bool write Tags"."NVH Operator Pass"."DataSocket Reference"."OnDataUpdated" format="%.0x"; "PLC bool write Tags"."NVH Operator Express Rollo Opened02"."DataSocket Reference"."OnStatusUpdated" format="%.0x"; "PLC bool write Tags"."NVH Operator Express Rollo Opened02"."DataSocket Reference"."OnDataUpdated" format="%.0x"; "PLC bool write Tags"."NVH Operator Express Rollo Closed01"."DataSocket Reference"."OnStatusUpdated" format="%.0x"; "PLC bool write Tags"."NVH Operator Express Rollo Closed01"."DataSocket Reference"."OnDataUpdated" format="%.0x"; "PLC bool write Tags"."NVH Operator Express Rollo Opened01"."DataSocket Reference"."OnStatusUpdated" format="%.0x"; "PLC bool write Tags"."NVH Operator Express Rollo Opened01"."DataSocket Reference"."OnDataUpdated" format="%.0x"; "PLC bool write Tags"."NVH Operator Express Glass Closed"."DataSocket Reference"."OnStatusUpdated" format="%.0x"; "PLC bool write Tags"."NVH Operator Express Glass Closed"."DataSocket Reference"."OnDataUpdated" format="%.0x"; "PLC bool write Tags"."NVH Operator Express Glass Opened"."DataSocket Reference"."OnStatusUpdated" format="%.0x"; "PLC bool write Tags"."NVH Operator Express Glass Opened"."DataSocket Reference"."OnDataUpdated" format="%.0x"; "PLC bool write Tags"."NVH Fail"."DataSocket Reference"."OnStatusUpdated" format="%.0x"; "PLC bool write Tags"."NVH Fail"."DataSocket Reference"."OnDataUpdated" format="%.0x"; "PLC bool write Tags"."NVH Pass"."DataSocket Reference"."OnStatusUpdated" format="%.0x"; "PLC bool write Tags"."NVH Pass"."DataSocket Reference"."OnDataUpdated" format="%.0x"; "PLC bool write Tags"."NVH SunRoof Stop"."DataSocket Reference"."OnStatusUpdated" format="%.0x"; "PLC bool write Tags"."NVH SunRoof Stop"."DataSocket Reference"."OnDataUpdated" format="%.0x"; "PLC bool write Tags"."NVH SunRoof Moving"."DataSocket Reference"."OnStatusUpdated" format="%.0x"; "PLC bool write Tags"."NVH SunRoof Moving"."DataSocket Reference"."OnDataUpdated" format="%.0x"; "PLC bool write Tags"."Extend Z LVDTS"."DataSocket Reference"."OnStatusUpdated" format="%.0x"; "PLC bool write Tags"."Extend Z LVDTS"."DataSocket Reference"."OnDataUpdated" format="%.0x"; "PLC bool write Tags"."Bad Frame Barcode"."DataSocket Reference"."OnStatusUpdated" format="%.0x"; "PLC bool write Tags"."Bad Frame Barcode"."DataSocket Reference"."OnDataUpdated" format="%.0x"; "PLC bool write Tags"."Good Frame Barcode"."DataSocket Reference"."OnStatusUpdated" format="%.0x"; "PLC bool write Tags"."Good Frame Barcode"."DataSocket Reference"."OnDataUpdated" format="%.0x"; "PLC bool write Tags"."AT VentPMACExtended"."DataSocket Reference"."OnStatusUpdated" format="%.0x"; "PLC bool write Tags"."AT VentPMACExtended"."DataSocket Reference"."OnDataUpdated" format="%.0x"; "PLC bool write Tags"."AT VentPMACHome"."DataSocket Reference"."OnStatusUpdated" format="%.0x"; "PLC bool write Tags"."AT VentPMACHome"."DataSocket Reference"."OnDataUpdated" format="%.0x"; "PLC bool write Tags"."control slide stop"."DataSocket Reference"."OnStatusUpdated" format="%.0x"; "PLC bool write Tags"."control slide stop"."DataSocket Reference"."OnDataUpdated" format="%.0x"; "PLC bool write Tags"."control slide start"."DataSocket Reference"."OnStatusUpdated" format="%.0x"; "PLC bool write Tags"."control slide start"."DataSocket Reference"."OnDataUpdated" format="%.0x"; "PLC bool write Tags"."ss servo close"."DataSocket Reference"."OnStatusUpdated" format="%.0x"; "PLC bool write Tags"."ss servo close"."DataSocket Reference"."OnDataUpdated" format="%.0x"; "PLC bool write Tags"."ss servo open"."DataSocket Reference"."OnStatusUpdated" format="%.0x"; "PLC bool write Tags"."ss servo open"."DataSocket Reference"."OnDataUpdated" format="%.0x"; "PLC bool write Tags"."Extend LVDT's"."DataSocket Reference"."OnStatusUpdated" format="%.0x"; "PLC bool write Tags"."Extend LVDT's"."DataSocket Reference"."OnDataUpdated" format="%.0x"; "PLC bool write Tags"."Retract LVDT's"."DataSocket Reference"."OnStatusUpdated" format="%.0x"; "PLC bool write Tags"."Retract LVDT's"."DataSocket Reference"."OnDataUpdated" format="%.0x"; "PLC bool write Tags"."Test Started"."DataSocket Reference"."OnStatusUpdated" format="%.0x"; "PLC bool write Tags"."Test Started"."DataSocket Reference"."OnDataUpdated" format="%.0x"; "PLC bool write Tags"."Test Complete Fail"."DataSocket Reference"."OnStatusUpdated" format="%.0x"; "PLC bool write Tags"."Test Complete Fail"."DataSocket Reference"."OnDataUpdated" format="%.0x"; "PLC bool write Tags"."Test Complete Pass"."DataSocket Reference"."OnStatusUpdated" format="%.0x"; "PLC bool write Tags"."Test Complete Pass"."DataSocket Reference"."OnDataUpdated" format="%.0x"; "PLC bool write Tags"."AT set wand home pos"."DataSocket Reference"."OnStatusUpdated" format="%.0x"; "PLC bool write Tags"."AT set wand home pos"."DataSocket Reference"."OnDataUpdated" format="%.0x"; "PLC bool write Tags"."AT set sunshade wand lower"."DataSocket Reference"."OnStatusUpdated" format="%.0x"; "PLC bool write Tags"."AT set sunshade wand lower"."DataSocket Reference"."OnDataUpdated" format="%.0x"; "PLC bool write Tags"."AT set glass wand lower"."DataSocket Reference"."OnStatusUpdated" format="%.0x"; "PLC bool write Tags"."AT set glass wand lower"."DataSocket Reference"."OnDataUpdated" format="%.0x"; "PLC boolean read Tags"."AT in sunshad wand up pos"."DataSocket Reference"."OnStatusUpdated" format="%.0x"; "PLC boolean read Tags"."AT in sunshad wand up pos"."DataSocket Reference"."OnDataUpdated" format="%.0x"; "PLC boolean read Tags"."AT in glass wand up pos"."DataSocket Reference"."OnStatusUpdated" format="%.0x"; "PLC boolean read Tags"."AT in glass wand up pos"."DataSocket Reference"."OnDataUpdated" format="%.0x"; "PLC boolean read Tags"."Finish Adjust LVDT"."DataSocket Reference"."OnStatusUpdated" format="%.0x"; "PLC boolean read Tags"."Finish Adjust LVDT"."DataSocket Reference"."OnDataUpdated" format="%.0x"; "PLC boolean read Tags"."Start Adjust LVDT"."DataSocket Reference"."OnStatusUpdated" format="%.0x"; "PLC boolean read Tags"."Start Adjust LVDT"."DataSocket Reference"."OnDataUpdated" format="%.0x"; "PLC boolean read Tags"."AT at vent ATS Home pos"."DataSocket Reference"."OnStatusUpdated" format="%.0x"; "PLC boolean read Tags"."AT at vent ATS Home pos"."DataSocket Reference"."OnDataUpdated" format="%.0x"; "PLC boolean read Tags"."AT at vent ATS test pos"."DataSocket Reference"."OnStatusUpdated" format="%.0x"; "PLC boolean read Tags"."AT at vent ATS test pos"."DataSocket Reference"."OnDataUpdated" format="%.0x"; "PLC boolean read Tags"."NVH Operator Re-do"."DataSocket Reference"."OnStatusUpdated" format="%.0x"; "PLC boolean read Tags"."NVH Operator Re-do"."DataSocket Reference"."OnDataUpdated" format="%.0x"; "PLC boolean read Tags"."NVH Operator Express Glass Vent Close"."DataSocket Reference"."OnStatusUpdated" format="%.0x"; "PLC boolean read Tags"."NVH Operator Express Glass Vent Close"."DataSocket Reference"."OnDataUpdated" format="%.0x"; "PLC boolean read Tags"."NVH Operator Express Glass vent Open"."DataSocket Reference"."OnStatusUpdated" format="%.0x"; "PLC boolean read Tags"."NVH Operator Express Glass vent Open"."DataSocket Reference"."OnDataUpdated" format="%.0x"; "PLC boolean read Tags"."windproof position"."DataSocket Reference"."OnStatusUpdated" format="%.0x"; "PLC boolean read Tags"."windproof position"."DataSocket Reference"."OnDataUpdated" format="%.0x"; "PLC boolean read Tags"."NVH Operator Check"."DataSocket Reference"."OnStatusUpdated" format="%.0x"; "PLC boolean read Tags"."NVH Operator Check"."DataSocket Reference"."OnDataUpdated" format="%.0x"; "PLC boolean read Tags"."NVH Operator Finish"."DataSocket Reference"."OnStatusUpdated" format="%.0x"; "PLC boolean read Tags"."NVH Operator Finish"."DataSocket Reference"."OnDataUpdated" format="%.0x"; "PLC boolean read Tags"."NVH Operator Glass Close Noise"."DataSocket Reference"."OnStatusUpdated" format="%.0x"; "PLC boolean read Tags"."NVH Operator Glass Close Noise"."DataSocket Reference"."OnDataUpdated" format="%.0x"; "PLC boolean read Tags"."NVH Operator Glass Open Noise"."DataSocket Reference"."OnStatusUpdated" format="%.0x"; "PLC boolean read Tags"."NVH Operator Glass Open Noise"."DataSocket Reference"."OnDataUpdated" format="%.0x"; "PLC boolean read Tags"."NVH Operator Sunshade Close Noise"."DataSocket Reference"."OnStatusUpdated" format="%.0x"; "PLC boolean read Tags"."NVH Operator Sunshade Close Noise"."DataSocket Reference"."OnDataUpdated" format="%.0x"; "PLC boolean read Tags"."NVH Operator Sunshade Open Noise"."DataSocket Reference"."OnStatusUpdated" format="%.0x"; "PLC boolean read Tags"."NVH Operator Sunshade Open Noise"."DataSocket Reference"."OnDataUpdated" format="%.0x"; "PLC boolean read Tags"."NVH Operator Vent Close Noise"."DataSocket Reference"."OnStatusUpdated" format="%.0x"; "PLC boolean read Tags"."NVH Operator Vent Close Noise"."DataSocket Reference"."OnDataUpdated" format="%.0x"; "PLC boolean read Tags"."NVH Operator Vent Open Noise"."DataSocket Reference"."OnStatusUpdated" format="%.0x"; "PLC boolean read Tags"."NVH Operator Vent Open Noise"."DataSocket Reference"."OnDataUpdated" format="%.0x"; "PLC boolean read Tags"."NVH Operator Express Rollo Close02"."DataSocket Reference"."OnStatusUpdated" format="%.0x"; "PLC boolean read Tags"."NVH Operator Express Rollo Close02"."DataSocket Reference"."OnDataUpdated" format="%.0x"; "PLC boolean read Tags"."NVH Operator Express Rollo Open02"."DataSocket Reference"."OnStatusUpdated" format="%.0x"; "PLC boolean read Tags"."NVH Operator Express Rollo Open02"."DataSocket Reference"."OnDataUpdated" format="%.0x"; "PLC boolean read Tags"."NVH Operator Express Rollo Close01"."DataSocket Reference"."OnStatusUpdated" format="%.0x"; "PLC boolean read Tags"."NVH Operator Express Rollo Close01"."DataSocket Reference"."OnDataUpdated" format="%.0x"; "PLC boolean read Tags"."NVH Operator Express Rollo Open01"."DataSocket Reference"."OnStatusUpdated" format="%.0x"; "PLC boolean read Tags"."NVH Operator Express Rollo Open01"."DataSocket Reference"."OnDataUpdated" format="%.0x"; "PLC boolean read Tags"."NVH Operator Express Glass Close"."DataSocket Reference"."OnStatusUpdated" format="%.0x"; "PLC boolean read Tags"."NVH Operator Express Glass Close"."DataSocket Reference"."OnDataUpdated" format="%.0x"; "PLC boolean read Tags"."NVH Operator Express Glass Open"."DataSocket Reference"."OnStatusUpdated" format="%.0x"; "PLC boolean read Tags"."NVH Operator Express Glass Open"."DataSocket Reference"."OnDataUpdated" format="%.0x"; "PLC boolean read Tags"."NVH Operator Fail"."DataSocket Reference"."OnStatusUpdated" format="%.0x"; "PLC boolean read Tags"."NVH Operator Fail"."DataSocket Reference"."OnDataUpdated" format="%.0x"; "PLC boolean read Tags"."NVH Operator Pass"."DataSocket Reference"."OnStatusUpdated" format="%.0x"; "PLC boolean read Tags"."NVH Operator Pass"."DataSocket Reference"."OnDataUpdated" format="%.0x"; "PLC boolean read Tags"."Z LVDTs Extended"."DataSocket Reference"."OnStatusUpdated" format="%.0x"; "PLC boolean read Tags"."Z LVDTs Extended"."DataSocket Reference"."OnDataUpdated" format="%.0x"; "PLC boolean read Tags"."Check Frame Barcode"."DataSocket Reference"."OnStatusUpdated" format="%.0x"; "PLC boolean read Tags"."Check Frame Barcode"."DataSocket Reference"."OnDataUpdated" format="%.0x"; "PLC boolean read Tags"."SS Barcode Scanner Bypassed"."DataSocket Reference"."OnStatusUpdated" format="%.0x"; "PLC boolean read Tags"."SS Barcode Scanner Bypassed"."DataSocket Reference"."OnDataUpdated" format="%.0x"; "PLC boolean read Tags"."AT VentPMACisExtend"."DataSocket Reference"."OnStatusUpdated" format="%.0x"; "PLC boolean read Tags"."AT VentPMACisExtend"."DataSocket Reference"."OnDataUpdated" format="%.0x"; "PLC boolean read Tags"."AT VentPMACatHome"."DataSocket Reference"."OnStatusUpdated" format="%.0x"; "PLC boolean read Tags"."AT VentPMACatHome"."DataSocket Reference"."OnDataUpdated" format="%.0x"; "PLC boolean read Tags"."wind deflector low speed pos"."DataSocket Reference"."OnStatusUpdated" format="%.0x"; "PLC boolean read Tags"."wind deflector low speed pos"."DataSocket Reference"."OnDataUpdated" format="%.0x"; "PLC boolean read Tags"."wind deflector high speed pos"."DataSocket Reference"."OnStatusUpdated" format="%.0x"; "PLC boolean read Tags"."wind deflector high speed pos"."DataSocket Reference"."OnDataUpdated" format="%.0x"; "PLC boolean read Tags"."control slide right over stroke"."DataSocket Reference"."OnStatusUpdated" format="%.0x"; "PLC boolean read Tags"."control slide right over stroke"."DataSocket Reference"."OnDataUpdated" format="%.0x"; "PLC boolean read Tags"."control slide right good"."DataSocket Reference"."OnStatusUpdated" format="%.0x"; "PLC boolean read Tags"."control slide right good"."DataSocket Reference"."OnDataUpdated" format="%.0x"; "PLC boolean read Tags"."control slide left over stroke"."DataSocket Reference"."OnStatusUpdated" format="%.0x"; "PLC boolean read Tags"."control slide left over stroke"."DataSocket Reference"."OnDataUpdated" format="%.0x"; "PLC boolean read Tags"."control slide left good"."DataSocket Reference"."OnStatusUpdated" format="%.0x"; "PLC boolean read Tags"."control slide left good"."DataSocket Reference"."OnDataUpdated" format="%.0x"; "PLC boolean read Tags"."control slide at home"."DataSocket Reference"."OnStatusUpdated" format="%.0x"; "PLC boolean read Tags"."control slide at home"."DataSocket Reference"."OnDataUpdated" format="%.0x"; "PLC boolean read Tags"."ss servo closing"."DataSocket Reference"."OnStatusUpdated" format="%.0x"; "PLC boolean read Tags"."ss servo closing"."DataSocket Reference"."OnDataUpdated" format="%.0x"; "PLC boolean read Tags"."ss servo opening"."DataSocket Reference"."OnStatusUpdated" format="%.0x"; "PLC boolean read Tags"."ss servo opening"."DataSocket Reference"."OnDataUpdated" format="%.0x"; "PLC boolean read Tags"."ss servo at close"."DataSocket Reference"."OnStatusUpdated" format="%.0x"; "PLC boolean read Tags"."ss servo at close"."DataSocket Reference"."OnDataUpdated" format="%.0x"; "PLC boolean read Tags"."ss servo at open"."DataSocket Reference"."OnStatusUpdated" format="%.0x"; "PLC boolean read Tags"."ss servo at open"."DataSocket Reference"."OnDataUpdated" format="%.0x"; "PLC boolean read Tags"."manual barcode print"."DataSocket Reference"."OnStatusUpdated" format="%.0x"; "PLC boolean read Tags"."manual barcode print"."DataSocket Reference"."OnDataUpdated" format="%.0x"; "PLC boolean read Tags"."LVDT's Retracted"."DataSocket Reference"."OnStatusUpdated" format="%.0x"; "PLC boolean read Tags"."LVDT's Retracted"."DataSocket Reference"."OnDataUpdated" format="%.0x"; "PLC boolean read Tags"."abort"."DataSocket Reference"."OnStatusUpdated" format="%.0x"; "PLC boolean read Tags"."abort"."DataSocket Reference"."OnDataUpdated" format="%.0x"; "PLC boolean read Tags"."start"."DataSocket Reference"."OnStatusUpdated" format="%.0x"; "PLC boolean read Tags"."start"."DataSocket Reference"."OnDataUpdated" format="%.0x"; "PLC boolean read Tags"."bolt check 8"."DataSocket Reference"."OnStatusUpdated" format="%.0x"; "PLC boolean read Tags"."bolt check 8"."DataSocket Reference"."OnDataUpdated" format="%.0x"; "PLC boolean read Tags"."bolt check 7"."DataSocket Reference"."OnStatusUpdated" format="%.0x"; "PLC boolean read Tags"."bolt check 7"."DataSocket Reference"."OnDataUpdated" format="%.0x"; "PLC boolean read Tags"."bolt check 6"."DataSocket Reference"."OnStatusUpdated" format="%.0x"; "PLC boolean read Tags"."bolt check 6"."DataSocket Reference"."OnDataUpdated" format="%.0x"; "PLC boolean read Tags"."bolt check 5"."DataSocket Reference"."OnStatusUpdated" format="%.0x"; "PLC boolean read Tags"."bolt check 5"."DataSocket Reference"."OnDataUpdated" format="%.0x"; "PLC boolean read Tags"."bolt check 4"."DataSocket Reference"."OnStatusUpdated" format="%.0x"; "PLC boolean read Tags"."bolt check 4"."DataSocket Reference"."OnDataUpdated" format="%.0x"; "PLC boolean read Tags"."bolt check 3"."DataSocket Reference"."OnStatusUpdated" format="%.0x"; "PLC boolean read Tags"."bolt check 3"."DataSocket Reference"."OnDataUpdated" format="%.0x"; "PLC boolean read Tags"."bolt check 2"."DataSocket Reference"."OnStatusUpdated" format="%.0x"; "PLC boolean read Tags"."bolt check 2"."DataSocket Reference"."OnDataUpdated" format="%.0x"; "PLC boolean read Tags"."bolt check 1"."DataSocket Reference"."OnStatusUpdated" format="%.0x"; "PLC boolean read Tags"."bolt check 1"."DataSocket Reference"."OnDataUpdated" format="%.0x"; "PLC boolean read Tags"."LVDT's Extended"."DataSocket Reference"."OnStatusUpdated" format="%.0x"; "PLC boolean read Tags"."LVDT's Extended"."DataSocket Reference"."OnDataUpdated" format="%.0x"; "PLC boolean read Tags"."AT in wand home pos"."DataSocket Reference"."OnStatusUpdated" format="%.0x"; "PLC boolean read Tags"."AT in wand home pos"."DataSocket Reference"."OnDataUpdated" format="%.0x"; "PLC boolean read Tags"."AT in sunshad wand lower pos"."DataSocket Reference"."OnStatusUpdated" format="%.0x"; "PLC boolean read Tags"."AT in sunshad wand lower pos"."DataSocket Reference"."OnDataUpdated" format="%.0x"; "PLC boolean read Tags"."AT in glass wand lower pos"."DataSocket Reference"."OnStatusUpdated" format="%.0x"; "PLC boolean read Tags"."AT in glass wand lower pos"."DataSocket Reference"."OnDataUpdated" format="%.0x"; "PLC boolean read Tags"."AT shade position"."DataSocket Reference"."OnStatusUpdated" format="%.0x"; "PLC boolean read Tags"."AT shade position"."DataSocket Reference"."OnDataUpdated" format="%.0x"; "PLC boolean read Tags"."AT glass position"."DataSocket Reference"."OnStatusUpdated" format="%.0x"; "PLC boolean read Tags"."AT glass position"."DataSocket Reference"."OnDataUpdated" format="%.0x"}, 8 "错误输入":errorcluster, 11 "Config Info":T1) -> (0 "错误输出":errorcluster, 3 "Config Info out":T1)   [LabVIEW 2018]
uses:
  Type Def's/Config Info.ctl
  02.Type Def's/plc comms params.ctl
  02.Type Def's/station plc read boolean tags.ctl
  05.UserVI's/type defs/plc path and tag.ctl
  <vilib>/Platform/dataskt.llb/DataSocket Reference Type.ctl
  02.Type Def's/station plc write boolean tags.ctl
  02.Type Def's/station plc read string tags.ctl
  02.Type Def's/station plc write string tags.ctl
panel:
  # "start/abort only used by barcode instance, since there are discrete signals for this in the other stations."
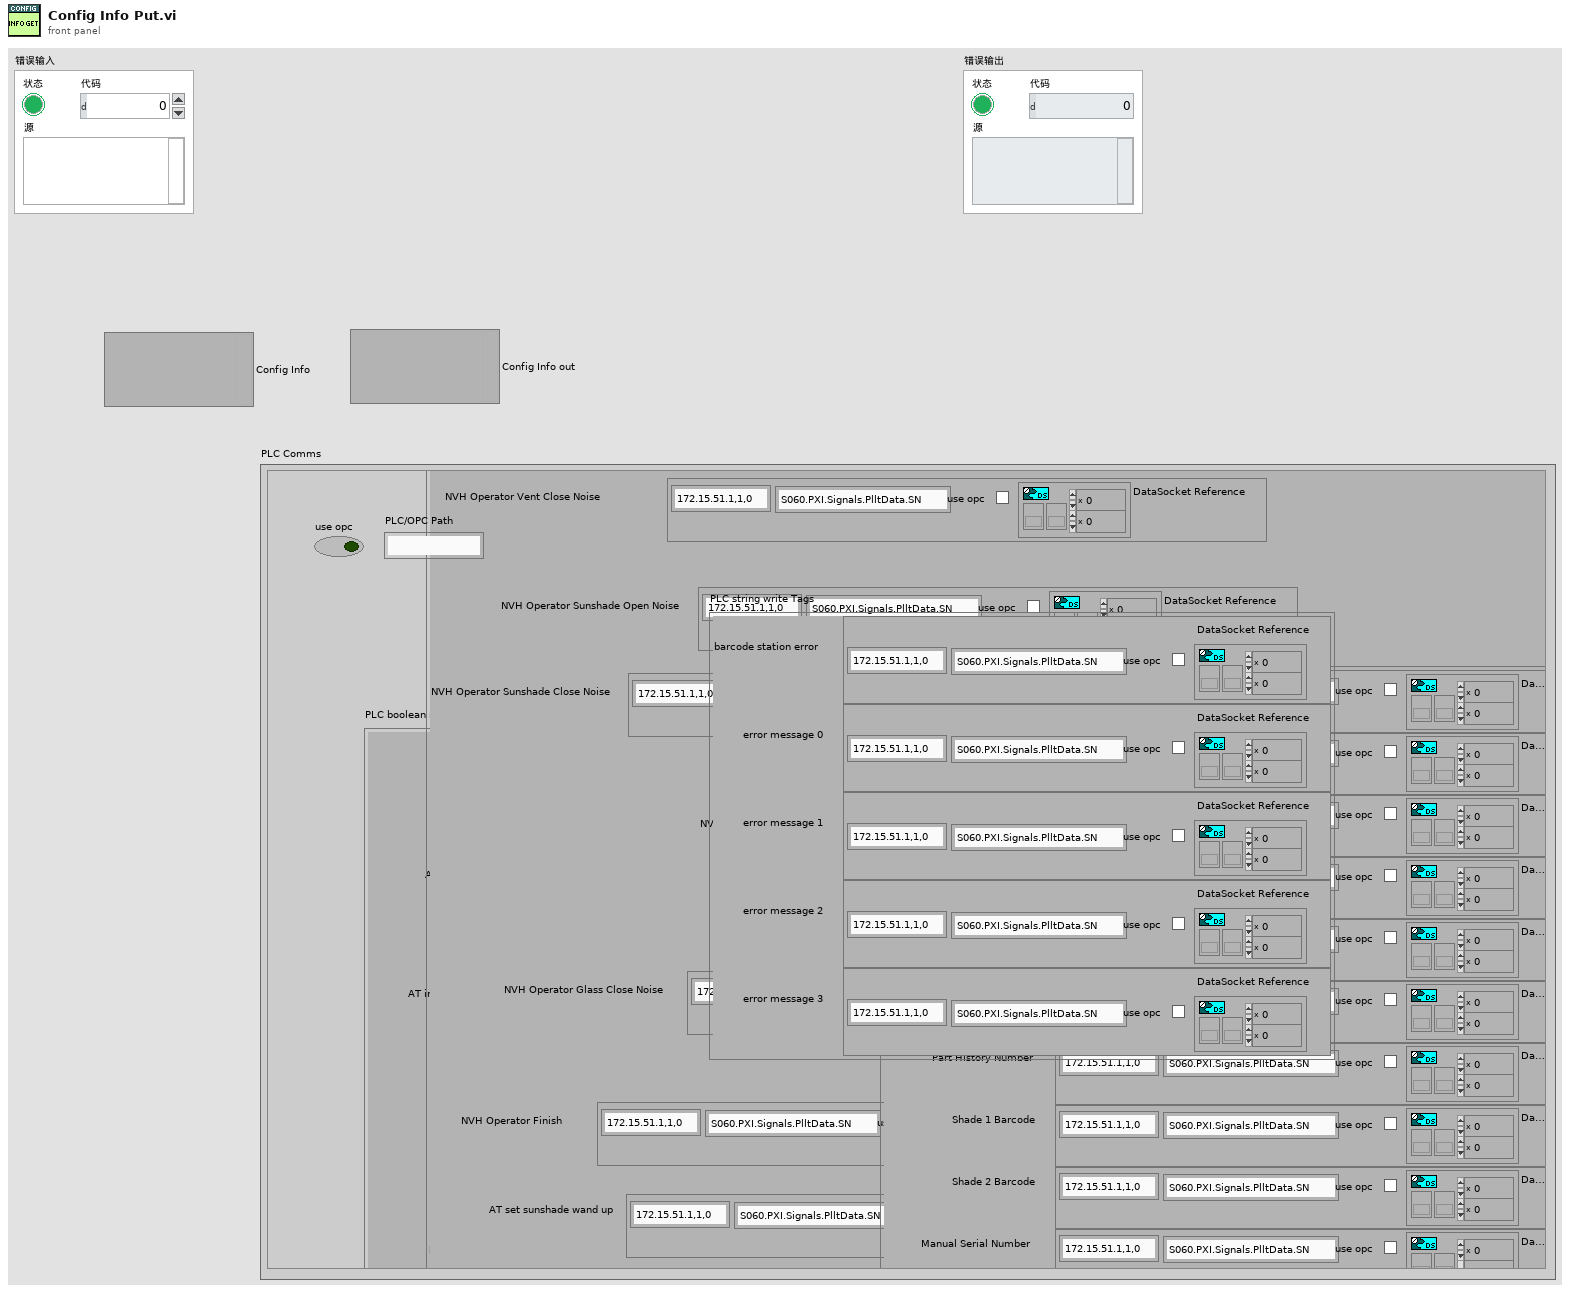
[diagram p1: front panel]
types:
  T1 = typedef "Config Info.ctl" = variant
  T2 = typedef "plc comms params.ctl" = cluster{"PLC boolean read Tags":T3, "PLC bool write Tags":T6, "PLC string read Tags":T7, "PLC string write Tags":T8, "use opc":bool, "PLC/OPC Path":string}
  T3 = typedef "station plc read boolean tags.ctl" = cluster{"AT glass position":T4, "AT shade position":T4, "AT in glass wand lower pos":T4, "AT in glass wand up pos":T4, "AT in sunshad wand lower pos":T4, "AT in sunshad wand up pos":T4, "AT in wand home pos":T4, "LVDT's Extended":T4, "bolt check 1":T4, "bolt check 2":T4, "bolt check 3":T4, "bolt check 4":T4, "bolt check 5":T4, "bolt check 6":T4, "bolt check 7":T4, "bolt check 8":T4, "start":T4, "abort":T4, "LVDT's Retracted":T4, "manual barcode print":T4, "ss servo at open":T4, "ss servo at close":T4, "ss servo opening":T4, "ss servo closing":T4, "control slide at home":T4, "control slide left good":T4, "control slide left over stroke":T4, "control slide right good":T4, "control slide right over stroke":T4, "wind deflector high speed pos":T4, "wind deflector low speed pos":T4, "AT VentPMACatHome":T4, "AT VentPMACisExtend":T4, "SS Barcode Scanner Bypassed":T4, "Check Frame Barcode":T4, "Z LVDTs Extended":T4, "NVH Operator Pass":T4, "NVH Operator Fail":T4, "NVH Operator Express Glass Open":T4, "NVH Operator Express Glass Close":T4, "NVH Operator Express Rollo Open01":T4, "NVH Operator Express Rollo Close01":T4, "NVH Operator Express Rollo Open02":T4, "NVH Operator Express Rollo Close02":T4, "NVH Operator Vent Open Noise":T4, "NVH Operator Vent Close Noise":T4, "NVH Operator Sunshade Open Noise":T4, "NVH Operator Sunshade Close Noise":T4, "NVH Operator Glass Open Noise":T4, "NVH Operator Glass Close Noise":T4, "NVH Operator Finish":T4, "NVH Operator Check":T4, "windproof position":T4, "NVH Operator Express Glass vent Open":T4, "NVH Operator Express Glass Vent Close":T4, "NVH Operator Re-do":T4, "AT at vent ATS test pos":T4, "AT at vent ATS Home pos":T4, "Start Adjust LVDT":T4, "Finish Adjust LVDT":T4}
  T4 = typedef "plc path and tag.ctl" = cluster{"Tag Name":string, "Network Path":string, "use opc":bool, "DataSocket Reference":T5}
  T5 = typedef "DataSocket Reference Type.ctl" = cluster{"CWDSLib._DCWDataSocket":refnum<k7>, "CWDSLib._DCWData":refnum<k7>, "OnDataUpdated":u32, "OnStatusUpdated":u32}
  T6 = typedef "station plc write boolean tags.ctl" = cluster{"AT set glass wand lower":T4, "AT set sunshade wand lower":T4, "AT set sunshade wand up":T4, "AT set glass wand up":T4, "AT set wand home pos":T4, "Test Complete Pass":T4, "Test Complete Fail":T4, "Test Started":T4, "Retract LVDT's":T4, "Extend LVDT's":T4, "ss servo open":T4, "ss servo close":T4, "control slide start":T4, "control slide stop":T4, "AT VentPMACHome":T4, "AT VentPMACExtended":T4, "Good Frame Barcode":T4, "Bad Frame Barcode":T4, "Extend Z LVDTS":T4, "NVH SunRoof Moving":T4, "NVH SunRoof Stop":T4, "NVH Pass":T4, "NVH Fail":T4, "NVH Operator Express Glass Opened":T4, "NVH Operator Express Glass Closed":T4, "NVH Operator Express Rollo Opened01":T4, "NVH Operator Express Rollo Closed01":T4, "NVH Operator Express Rollo Opened02":T4, "NVH Operator Pass":T4, "NVH Operator Fail":T4, "NVH Operator Check":T4, "NVH Operator Vent Open Noise":T4, "NVH Operator Vent Close Noise":T4, "NVH Operator Sunshade Open Noise":T4, "NVH Operator Sunshade Close Noise":T4, "NVH Operator Glass Open Noise":T4, "NVH Operator Glass Close Noise":T4, "NVH Operator Finish":T4, "Barcode01 OK":T4, "Barcode02 OK":T4, "AT set to Vent ATS Test Pos":T4, "AT set to Vent ATS Home Pos":T4, "Move LVDT Adjust Station":T4}
  T7 = typedef "station plc read string tags.ctl" = cluster{"Serial Number":T4, "Pallet Number":T4, "Inalfa Part Number":T4, "Shade Color":T4, "Model Type":T4, "Customer Number":T4, "Part History Number":T4, "Shade 1 Barcode":T4, "Shade 2 Barcode":T4, "Manual Serial Number":T4, "Manual Inalfa Part Number":T4, "Manual Shade Color":T4, "Manual Model Type":T4, "Manual Customer Number":T4, "Manual Part History Number":T4}
  T8 = typedef "station plc write string tags.ctl" = cluster{"barcode station error":T4, "error message 0":T4, "error message 1":T4, "error message 2":T4, "error message 3":T4}
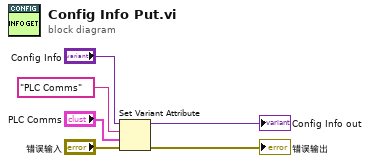
[diagram p0: block diagram]
diagram:
  n1 = Set Variant Attribute(Variant="Config Info", name="PLC Comms" ("名称"), value="PLC Comms", error in="错误输入") -> (Variant out=→"Config Info out":T1, error out=→"错误输出":errorcluster)  [unwired: 1 out]
